vi "Get Initial Stock Levels.vi"() -> (2 "Stock":T1[](array[typedef]), 3 "Stock file path":path)   [LabVIEW 2020, in "Stock.lvlib"]
uses:
  Stock.lvlib
  Products.ctl
  <vilib>/Utility/xml.llb/Read From XML File(string).vi
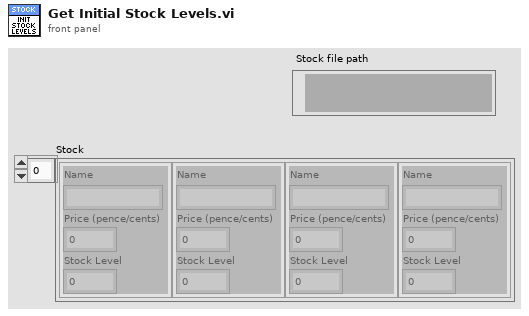
[diagram p1: front panel]
types:
  T1 = typedef "Stock.lvlib/Products.ctl" = cluster{"Name":string, "Price (pence/cents)":u32, "Stock Level":u32}
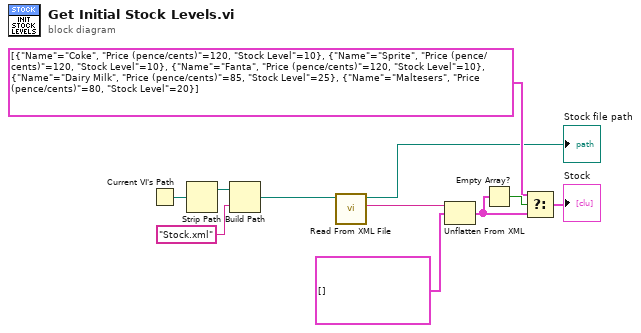
[diagram p0: block diagram]
diagram:
  n1 = Current VI's Path() -> (path=w9:path)
  n2 = Strip Path(path=w9) -> (stripped path=w8:path)  [unwired: 1 out]
  n3 = Build Path(base path=w8, name or relative path="Stock.xml") -> (appended path=w6:path)
  n4 = call-poly <vilib>:"Read From XML File.vi"("XML File Path"=w6) -> ("XML Elements"=w11:string, "XML File Path(duplicate)"=→"Stock file path":path)  [unwired: 8 in, 1 out]
  n5 = Unflatten From XML(xml string=w11, type=T1[] [] ("Stock")) -> (value=w3:T1[])  [unwired: 1 in, 1 out]
  n6 = Empty Array?(array=w3) -> (empty?=w5:bool)
  n7 = Select(t=T1[] [{"Name"="Coke", "Price (pence/cents)"=120, "Stock Level"=10}, {"Name"="Sprite", "Price (pence/cents)"=120, "Stock Level"=10}, {"Name"="Fanta", "Price (pence/cents)"=120, "Stock Level"=10}, {"Name"="Dairy Milk", "Price (pence/cents)"=85, "Stock Level"=25}, {"Name"="Maltesers", "Price (pence/cents)"=80, "Stock Level"=20}] ("Stock"), s=w5, f=w3) -> (s? t:f=→"Stock":T1[])
